vi "Glass Heater Accuracy.vi"() -> ()   [LabVIEW 2017]
uses:
  Shared Components/Gantry Class/Type Definitions/Virtual Modes.ctl
  Shared Components/Gantry Class/Type Definitions/Init_Modes.ctl
  Shared Components/Utils/Type Definitions/Object Types.ctl
  Shared Components/Config Manager Class/Type Definitions/Camera Enum.ctl
  Shared Components/Gantry Class/Gantry Class.lvclass
  Shared Components/Vec3d Class/Vec3d Class.lvclass
panel:
  in  "Results Folder":path=path "C:/Users/Admin/Gantry Purdue/pixel-gantry-control/Results"
  out "Iteration Number":i32
  in  "Virtual Mode":T1=enum."Virtual"
  in  "stop":bool
  out "Image":T2(plugin-control)
  out "error out":errorcluster
  in  "Config Folder":path=path "C:/Users/Admin/Gantry Purdue/pixel-gantry-control/Config"
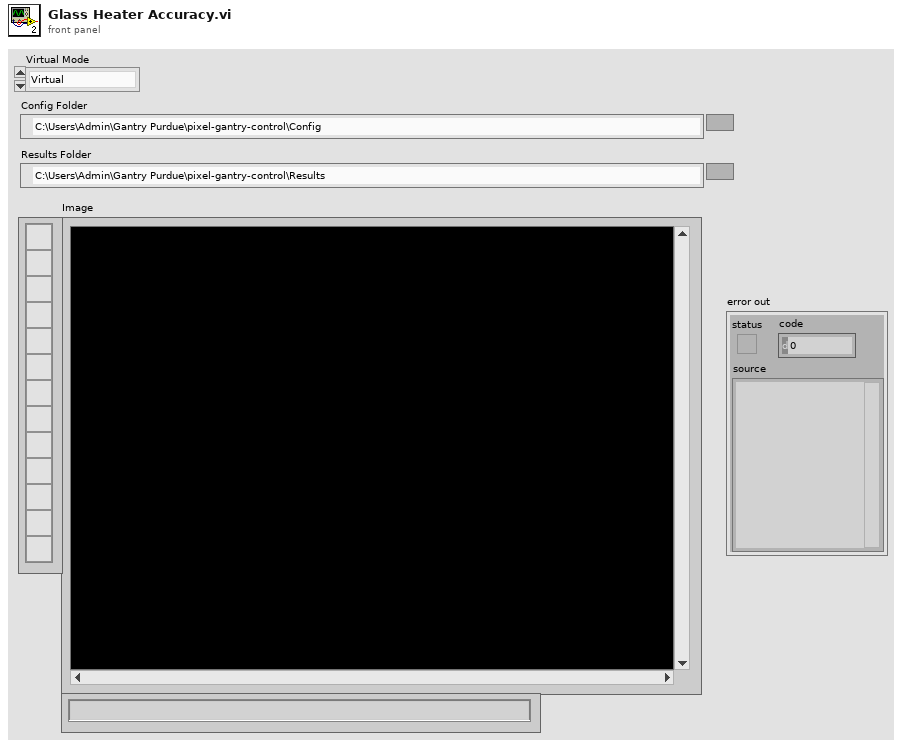
[diagram p1: front panel]
types:
  T1 = typedef "Virtual Modes.ctl" = enum16{"Nonvirtual", "Pseudovirtual", "Virtual"}
  T2 = typedef "IMAQ Image.ctl" = refnum<image>
  T3 = typedef "Init_Modes.ctl" = enum16{"Full", "Robot Only", "Dispenser Only", "Cameras Only", "Robot and Cameras", "Robot and Cameras and Dispenser", "Manifold Only"}
  T4 = typedef "Object Types.ctl" = enum16{"HDI", "Glass Piece", "Other"}
  T5 = typedef "Camera Enum.ctl" = enum16{"GANTRY HEAD", "NEEDLE CALIBRATION X", "NEEDLE CALIBRATION Y", "STAND CAMERA", "SIMRAN WEBCAM"}
  T6 = typedef "Physical Image.ctl" = cluster{"Image Position":refnum<class "Vec3d Class.lvclass">, "Image Reference":T2, "Field of View":cluster{"x(mm)":dbl, "y(mm)":dbl}}
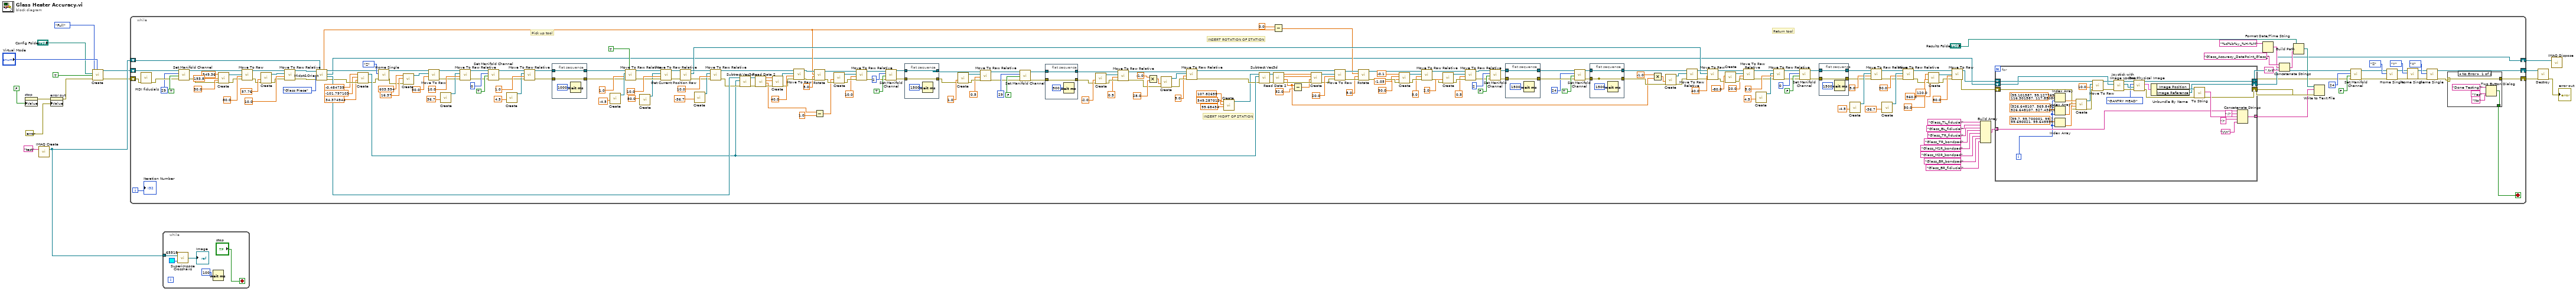
[diagram p0: block diagram]
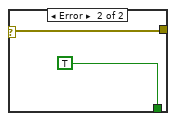
[diagram p2: hidden frame]
diagram:
  n1 = property on="stop" class="Bool (strict)"("Value"=FALSE) -> (error out=w14:errorcluster)  [unwired: 2 in, 1 out]
  n2 = call "IMAQ Create"("Image Name"="test") -> ("New Image"=w11:T2)  [unwired: 4 in, 1 out]
  n3 = property on="error out" class="Clust (strict)"(error in=w14, "Value"=errorcluster {"status"=FALSE, "code"=0, "source"=""} ("error in (no error)")) -> (error out=w9:errorcluster)  [unwired: 1 in, 1 out]
  n4 = call "Create.vi"("Virtual Mode"="Virtual Mode", "error in"=w9, "HOME?"=TRUE, "Config Folder"="Config Folder", "Init Mode"=Init_Modes."Full") -> ("error out"=w6:errorcluster, "Gantry out"=w5:refnum<class "Gantry Class.lvclass">)  [unwired: 5 in]
  n5 = while {
    shift-right: [w83] -> w3
    shift-left: w11 -> [w104]
    shift-right: [w106] -> w2
    shift-left: w5 -> [w140]
    shift-right: [w105] -> w1
    shift-left: w6 -> [w145]
    i -> [w142]
    stop <- w143 stop-if-true
    # "INSERT ROTATION OF STATION"
    # "INSERT MIDPT OF STATION"
    # "Pick up tool"
    # "Return tool"
    n6 = call "HDI fiducials"("error in (no error)"=w145) -> ("error out"=w138:errorcluster)  [unwired: 17 in, 1 out]
    n7 = call-dynamic "Set Manifold Channel.vi"("error in"=w138, "On/Off"=TRUE, "Manifold Channel"=29, "Gantry in"=w140) -> ("error out"=w137:errorcluster, "Gantry out"=w139:refnum<class "Gantry Class.lvclass">)  [unwired: 6 in]
    n8 = call "Create.vi"("error in"=w137, "Z"=30.0, "Y"=193.8, "X"=549.36) -> ("error out"=w225:errorcluster, "Vec3d Class out"=w258:refnum<class "Vec3d Class.lvclass">)  [unwired: 6 in]
    n9 = call-dynamic "Move To Raw.vi"("error in"=w225, "Speed"=80.0, "Destination"=w258, "Gantry in"=w139) -> ("error out"=w75:errorcluster, "Gantry out"=w80:refnum<class "Gantry Class.lvclass">)  [unwired: 6 in]
    n10 = call "Create.vi"("error in"=w75, "Z"=57.76) -> ("error out"=w74:errorcluster, "Vec3d Class out"=w81:refnum<class "Vec3d Class.lvclass">)  [unwired: 8 in]
    n11 = call-dynamic "Move To Raw Relative.vi"("error in"=w74, "Speed(mm/s)"=10.0, "Delta"=w81, "Gantry in"=w80) -> ("error out"=w78:errorcluster, "Gantry out"=w79:refnum<class "Gantry Class.lvclass">)  [unwired: 6 in]
    n12 = call-dynamic "Midpt&Orient.vi"("error in (no error)"=w78, "Enum"=Object_Types."Glass Piece", "Image In"=w104, "Gantry Class in"=w79) -> ("error out"=w158:errorcluster, "Midpoint"=w223:refnum<class "Vec3d Class.lvclass">, "Image Out"=w24:T2, "Gantry Class out"=w150:refnum<class "Gantry Class.lvclass">, "Orientation"=w147:dbl)  [unwired: 3 in]
    n13 = call "Create.vi"("error in"=w158, "Z"=34.374944 ("Y"), "Y"=-101.797103, "X"=-0.484739) -> ("error out"=w151:errorcluster, "Vec3d Class out"=w196:refnum<class "Vec3d Class.lvclass">)  [unwired: 6 in]
    n14 = call-dynamic "Home Single.vi"("error in"=w151, "Axis"=enum16{"X", "Y", "Z", "U"}."Z", "Gantry in"=w150) -> ("error out"=w148:errorcluster, "Gantry out"=w149:refnum<class "Gantry Class.lvclass">)  [unwired: 7 in]
    n15 = call "Create.vi"("error in"=w148, "Y"=16.37, "X"=603.594) -> ("Vec3d Class out"=w274:refnum<class "Vec3d Class.lvclass">)  [unwired: 7 in, 1 out]
    n16 = call-dynamic "Move To Raw.vi"("Speed"=50.0 ("Speed(mm/s)"), "Destination"=w274, "Gantry in"=w149) -> ("error out"=w170:errorcluster, "Gantry out"=w171:refnum<class "Gantry Class.lvclass">)  [unwired: 7 in]
    n17 = call "Create.vi"("Z"=36.7) -> ("Vec3d Class out"=w172:refnum<class "Vec3d Class.lvclass">)  [unwired: 9 in, 1 out]
    n18 = call-dynamic "Move To Raw Relative.vi"("error in"=w170, "Speed(mm/s)"=10.0, "Delta"=w172, "Gantry in"=w171) -> ("error out"=w64:errorcluster, "Gantry out"=w63:refnum<class "Gantry Class.lvclass">)  [unwired: 6 in]
    n19 = call-dynamic "Set Manifold Channel.vi"("error in"=w64, "On/Off"=TRUE, "Manifold Channel"=0, "Gantry in"=w63) -> ("error out"=w66:errorcluster, "Gantry out"=w68:refnum<class "Gantry Class.lvclass">)  [unwired: 6 in]
    n20 = call "Create.vi"("Z"=4.5) -> ("Vec3d Class out"=w69:refnum<class "Vec3d Class.lvclass">)  [unwired: 9 in, 1 out]
    n21 = call-dynamic "Move To Raw Relative.vi"("error in"=w66, "Speed(mm/s)"=1.0, "Delta"=w69, "Gantry in"=w68) -> ("error out"=w65:errorcluster, "Gantry out"=w67:refnum<class "Gantry Class.lvclass">)  [unwired: 6 in]
    n22 = flat-sequence {
      tunnel: w67 -> [w300]
      tunnel: [w300] -> w232
      tunnel: w65 -> [w298]
      tunnel: [w298] -> w231
      frame #0 {
        n23 = Wait (ms)(milliseconds to wait=u32 1000) -> ()  [unwired: 1 out]
      }
    }
    n24 = call "Create.vi"("Z"=-4.5) -> ("Vec3d Class out"=w269:refnum<class "Vec3d Class.lvclass">)  [unwired: 9 in, 1 out]
    n25 = call-dynamic "Move To Raw Relative.vi"("Wait?"=TRUE, "error in"=w231, "Speed(mm/s)"=1.0, "Delta"=w269, "Gantry in"=w232) -> ("error out"=w264:errorcluster, "Gantry out"=w265:refnum<class "Gantry Class.lvclass">)  [unwired: 5 in]
    n26 = call "Create.vi"("Y"=80.0 ("Z")) -> ("Vec3d Class out"=w263:refnum<class "Vec3d Class.lvclass">)  [unwired: 9 in, 1 out]
    n27 = call-dynamic "Move To Raw Relative.vi"("error in"=w264, "Speed(mm/s)"=10.0, "Delta"=w263, "Gantry in"=w265) -> ("error out"=w251:errorcluster, "Gantry out"=w253:refnum<class "Gantry Class.lvclass">)  [unwired: 6 in]
    n28 = call-dynamic "Get Current Position Raw.vi"("error in"=w251, "Gantry in"=w253) -> ("error out"=w250:errorcluster, "Vec3d Class out"=w187:refnum<class "Vec3d Class.lvclass">, "Gantry out"=w252:refnum<class "Gantry Class.lvclass">)  [unwired: 7 in]
    n29 = call "Create.vi"("Z"=-36.7) -> ("Vec3d Class out"=w259:refnum<class "Vec3d Class.lvclass">)  [unwired: 9 in, 1 out]
    n30 = call-dynamic "Move To Raw Relative.vi"("error in"=w250, "Speed(mm/s)"=10.0, "Delta"=w259, "Gantry in"=w252) -> ("error out"=w217:errorcluster, "Gantry out"=w215:refnum<class "Gantry Class.lvclass">)  [unwired: 6 in]
    n31 = call "Subtract Vec3d.vi"("error in (no error)"=w217, "Vec3d in 2"=w196, "Vec3d in 1"=w223) -> ("error out"=w219:errorcluster, "Vec3d Class out"=w176:refnum<class "Vec3d Class.lvclass">)  [unwired: 7 in]
    n32 = call-dynamic "Read Data 2.vi"("error in"=w219, "Vec3d in"=w176) -> ("error out"=w218:errorcluster, "Z"=w51:dbl, "Y"=w221:dbl, "X"=w222:dbl)  [unwired: 6 in]
    n33 = call "Create.vi"("error in"=w218, "Y"=w221, "X"=w222) -> ("error out"=w216:errorcluster, "Vec3d Class out"=w175:refnum<class "Vec3d Class.lvclass">)  [unwired: 7 in]
    n34 = call-dynamic "Move To Raw.vi"("error in"=w216, "Speed"=40.0, "Destination"=w175, "Gantry in"=w215) -> ("error out"=w186:errorcluster, "Gantry out"=w185:refnum<class "Gantry Class.lvclass">)  [unwired: 6 in]
    n35 = call-dynamic "Rotate.vi"("error in"=w186, "speed(deg/s)"=5.0, "distance(deg)"=w147, "Gantry in"=w185) -> ("error out"=w183:errorcluster, "Gantry out"=w184:refnum<class "Gantry Class.lvclass">)  [unwired: 6 in]
    n36 = Subtract(x=w51, y=1.0) -> (x-y=w50:dbl)
    n37 = call "Create.vi"("error in"=w183, "Z"=w50) -> ("error out"=w214:errorcluster, "Vec3d Class out"=w220:refnum<class "Vec3d Class.lvclass">)  [unwired: 8 in]
    n38 = call-dynamic "Move To Raw Relative.vi"("error in"=w214, "Speed(mm/s)"=10.0, "Delta"=w220, "Gantry in"=w184) -> ("error out"=w58:errorcluster, "Gantry out"=w57:refnum<class "Gantry Class.lvclass">)  [unwired: 6 in]
    n39 = call-dynamic "Set Manifold Channel.vi"("error in"=w58, "On/Off"=TRUE, "Manifold Channel"=2, "Gantry in"=w57) -> ("error out"=w60:errorcluster, "Gantry out"=w61:refnum<class "Gantry Class.lvclass">)  [unwired: 6 in]
    n40 = flat-sequence {
      tunnel: w61 -> [w278]
      tunnel: [w278] -> w53
      tunnel: w60 -> [w276]
      tunnel: [w276] -> w46
      frame #0 {
        n41 = Wait (ms)(milliseconds to wait=u32 1500) -> ()  [unwired: 1 out]
      }
    }
    n42 = call "Create.vi"("error in"=w46, "Z"=1.0 ("y")) -> ("error out"=w55:errorcluster, "Vec3d Class out"=w56:refnum<class "Vec3d Class.lvclass">)  [unwired: 8 in]
    n43 = call-dynamic "Move To Raw Relative.vi"("error in"=w55, "Speed(mm/s)"=0.5, "Delta"=w56, "Gantry in"=w53) -> ("error out"=w47:errorcluster, "Gantry out"=w48:refnum<class "Gantry Class.lvclass">)  [unwired: 6 in]
    n44 = call-dynamic "Set Manifold Channel.vi"("error in"=w47, "On/Off"=FALSE, "Manifold Channel"=29, "Gantry in"=w48) -> ("error out"=w133:errorcluster, "Gantry out"=w132:refnum<class "Gantry Class.lvclass">)  [unwired: 6 in]
    n45 = flat-sequence {
      tunnel: w132 -> [w284]
      tunnel: [w284] -> w41
      tunnel: w133 -> [w282]
      tunnel: [w282] -> w40
      frame #0 {
        n46 = Wait (ms)(milliseconds to wait=u32 500) -> ()  [unwired: 1 out]
      }
    }
    n47 = call "Create.vi"("error in"=w40, "Z"=-2.0 ("y")) -> ("error out"=w44:errorcluster, "Vec3d Class out"=w45:refnum<class "Vec3d Class.lvclass">)  [unwired: 8 in]
    n48 = call-dynamic "Move To Raw Relative.vi"("error in"=w44, "Speed(mm/s)"=0.5, "Delta"=w45, "Gantry in"=w41) -> ("error out"=w38:errorcluster, "Gantry out"=w39:refnum<class "Gantry Class.lvclass">)  [unwired: 6 in]
    n49 = Multiply(x=-1.0, y=28.0) -> (x*y=w256:dbl)
    n50 = call "Create.vi"("error in"=w38, "Z"=w256) -> ("error out"=w254:errorcluster, "Vec3d Class out"=w255:refnum<class "Vec3d Class.lvclass">)  [unwired: 8 in]
    n51 = call-dynamic "Move To Raw Relative.vi"("error in"=w254, "Speed(mm/s)"=5.0, "Delta"=w255, "Gantry in"=w39) -> ("error out"=w192:errorcluster, "Gantry out"=w193:refnum<class "Gantry Class.lvclass">)  [unwired: 6 in]
    n52 = call "Create.vi"("Z"=99.68434, "Y"=549.287012, "X"=107.82655) -> ("Vec3d Class out"=w103:refnum<class "Vec3d Class.lvclass">)  [unwired: 7 in, 1 out]
    n53 = call "Subtract Vec3d.vi"("error in (no error)"=w192, "Vec3d in 2"=w196, "Vec3d in 1"=w103) -> ("error out"=w203:errorcluster, "Vec3d Class out"=w206:refnum<class "Vec3d Class.lvclass">)  [unwired: 7 in]
    n54 = Subtract(x=0.0, y=w147) -> (x-y=w146:dbl)
    n55 = call-dynamic "Read Data 2.vi"("error in"=w203, "Vec3d in"=w206) -> ("error out"=w202:errorcluster, "Z"=w94:dbl, "Y"=w207:dbl, "X"=w208:dbl)  [unwired: 6 in]
    n56 = Subtract(x=w94, y=32.0) -> (x-y=w93:dbl)
    n57 = call "Create.vi"("error in"=w202, "Z"=w93, "Y"=w207, "X"=w208) -> ("error out"=w201:errorcluster, "Vec3d Class out"=w205:refnum<class "Vec3d Class.lvclass">)  [unwired: 6 in]
    n58 = call-dynamic "Move To Raw.vi"("error in"=w201, "Speed"=20.0, "Destination"=w205, "Gantry in"=w193) -> ("error out"=w180:errorcluster, "Gantry out"=w181:refnum<class "Gantry Class.lvclass">)  [unwired: 6 in]
    n59 = call-dynamic "Rotate.vi"("error in"=w180, "speed(deg/s)"=5.0, "distance(deg)"=w146, "Gantry in"=w181) -> ("error out"=w179:errorcluster, "Gantry out"=w178:refnum<class "Gantry Class.lvclass">)  [unwired: 6 in]
    n60 = call "Create.vi"("error in"=w179, "Z"=30.0, "Y"=-1.05, "X"=-0.1) -> ("error out"=w200:errorcluster, "Vec3d Class out"=w204:refnum<class "Vec3d Class.lvclass">)  [unwired: 6 in]
    n61 = call-dynamic "Move To Raw Relative.vi"("error in"=w200, "Speed(mm/s)"=5.0, "Delta"=w204, "Gantry in"=w178) -> ("error out"=w32:errorcluster, "Gantry out"=w33:refnum<class "Gantry Class.lvclass">)  [unwired: 6 in]
    n62 = call "Create.vi"("error in"=w32, "Z"=2.0) -> ("error out"=w36:errorcluster, "Vec3d Class out"=w37:refnum<class "Vec3d Class.lvclass">)  [unwired: 8 in]
    n63 = call-dynamic "Move To Raw Relative.vi"("error in"=w36, "Speed(mm/s)"=0.5, "Delta"=w37, "Gantry in"=w33) -> ("error out"=w31:errorcluster, "Gantry out"=w30:refnum<class "Gantry Class.lvclass">)  [unwired: 6 in]
    n64 = call-dynamic "Set Manifold Channel.vi"("error in"=w31, "On/Off"=FALSE, "Manifold Channel"=2, "Gantry in"=w30) -> ("error out"=w195:errorcluster, "Gantry out"=w194:refnum<class "Gantry Class.lvclass">)  [unwired: 6 in]
    n65 = flat-sequence {
      tunnel: w194 -> [w294]
      tunnel: [w294] -> w128
      tunnel: w195 -> [w292]
      tunnel: [w292] -> w125
      frame #0 {
        n66 = Wait (ms)(milliseconds to wait=u32 1500) -> ()  [unwired: 1 out]
      }
    }
    n67 = call-dynamic "Set Manifold Channel.vi"("error in"=w125, "On/Off"=TRUE, "Manifold Channel"=24, "Gantry in"=w128) -> ("error out"=w130:errorcluster, "Gantry out"=w129:refnum<class "Gantry Class.lvclass">)  [unwired: 6 in]
    n68 = flat-sequence {
      tunnel: w129 -> [w281]
      tunnel: [w281] -> w127
      tunnel: w130 -> [w279]
      tunnel: [w279] -> _
      tunnel: [w279] -> w126
      frame #0 {
        n69 = Wait (ms)(milliseconds to wait=u32 1500) -> ()  [unwired: 1 out]
      }
    }
    n70 = Multiply(x=-1.0, y=w94) -> (x*y=w210:dbl)
    n71 = call "Create.vi"("error in"=w126, "Z"=w210) -> ("error out"=w191:errorcluster, "Vec3d Class out"=w188:refnum<class "Vec3d Class.lvclass">)  [unwired: 8 in]
    n72 = call-dynamic "Move To Raw Relative.vi"("error in"=w191, "Delta"=w188, "Gantry in"=w127) -> ("error out"=w189:errorcluster, "Gantry out"=w190:refnum<class "Gantry Class.lvclass">)  [unwired: 7 in]
    n73 = call-dynamic "Move To Raw.vi"("error in"=w189, "Speed"=40.0, "Destination"=w187, "Gantry in"=w190) -> ("error out"=w161:errorcluster, "Gantry out"=w169:refnum<class "Gantry Class.lvclass">)  [unwired: 6 in]
    n74 = call "Create.vi"("error in"=w161, "Y"=-80.0) -> ("error out"=w248:errorcluster, "Vec3d Class out"=w233:refnum<class "Vec3d Class.lvclass">)  [unwired: 8 in]
    n75 = call-dynamic "Move To Raw Relative.vi"("error in"=w248, "Speed(mm/s)"=20.0, "Delta"=w233, "Gantry in"=w169) -> ("error out"=w234:errorcluster, "Gantry out"=w235:refnum<class "Gantry Class.lvclass">)  [unwired: 6 in]
    n76 = call "Create.vi"("Z"=4.5) -> ("Vec3d Class out"=w241:refnum<class "Vec3d Class.lvclass">)  [unwired: 9 in, 1 out]
    n77 = call-dynamic "Move To Raw Relative.vi"("error in"=w234, "Speed(mm/s)"=5.0, "Delta"=w241, "Gantry in"=w235) -> ("error out"=w239:errorcluster, "Gantry out"=w240:refnum<class "Gantry Class.lvclass">)  [unwired: 6 in]
    n78 = call-dynamic "Set Manifold Channel.vi"("error in"=w239, "On/Off"=FALSE, "Manifold Channel"=0, "Gantry in"=w240) -> ("error out"=w228:errorcluster, "Gantry out"=w230:refnum<class "Gantry Class.lvclass">)  [unwired: 6 in]
    n79 = flat-sequence {
      tunnel: w230 -> [w297]
      tunnel: [w297] -> w229
      tunnel: w228 -> [w295]
      tunnel: [w295] -> w227
      frame #0 {
        n80 = Wait (ms)(milliseconds to wait=u32 1500) -> ()  [unwired: 1 out]
      }
    }
    n81 = call "Create.vi"("Z"=-4.5) -> ("Vec3d Class out"=w237:refnum<class "Vec3d Class.lvclass">)  [unwired: 9 in, 1 out]
    n82 = call-dynamic "Move To Raw Relative.vi"("error in"=w227, "Speed(mm/s)"=5.0, "Delta"=w237, "Gantry in"=w229) -> ("error out"=w116:errorcluster, "Gantry out"=w117:refnum<class "Gantry Class.lvclass">)  [unwired: 6 in]
    n83 = call "Create.vi"("Z"=-36.7) -> ("Vec3d Class out"=w119:refnum<class "Vec3d Class.lvclass">)  [unwired: 9 in, 1 out]
    n84 = call-dynamic "Move To Raw Relative.vi"("error in"=w116, "Speed(mm/s)"=50.0, "Delta"=w119, "Gantry in"=w117) -> ("error out"=w107:errorcluster, "Gantry out"=w108:refnum<class "Gantry Class.lvclass">)  [unwired: 6 in]
    n85 = call "Create.vi"("error in"=w107, "Z"=30.0, "Y"=560.0, "X"=120.0) -> ("error out"=w111:errorcluster, "Vec3d Class out"=w113:refnum<class "Vec3d Class.lvclass">)  [unwired: 6 in]
    n86 = call-dynamic "Move To Raw.vi"("error in"=w111, "Speed"=80.0, "Destination"=w113, "Gantry in"=w108) -> ("error out"=w25:errorcluster, "Gantry out"=w26:refnum<class "Gantry Class.lvclass">)  [unwired: 6 in]
    n87 = Build Array("Glass_TL_fiducial" ("string"), "Glass_BL_fidiucial" ("string"), "Glass_TR_fiducial" ("string"), "Glass_TR_bondpad" ("string"), "Glass_M1R_bondpad" ("string"), "Glass_M2R_bondpad" ("string"), "Glass_BR_bondpad" ("string"), "Glass_BR_fidiucial" ("string")) -> (w27:string[])
    n88 = for {
      tunnel: [w324] -> w23 mode=indexing
      shift-right: [w325] -> w85
      shift-left: w25 -> [w301]
      shift-right: [w323] -> w84
      shift-left: w26 -> [w318]
      shift-right: [w319] -> w83
      shift-left: w24 -> [w307]
      tunnel: w27 -> [w303] mode=indexing
      i -> [w302]
      n89 = Index Array(array=dbl[] [99.101587, 99.127769, 116.301587, 117.850807, 117.863228, 117.862293, 117.873652, 116.327769], index=w302) -> (element=w315:dbl)
      n90 = Index Array(array=dbl[] [526.648107, 569.84924, 526.648107, 527.43622, 547.203352, 549.29103, 569.056008, 569.84924], index=w302) -> (element=w314:dbl)
      n91 = Index Array(array=dbl[] [99.7, 99.700001, 99.7, 99.690021, 99.649999, 99.684328, 99.645157, 99.700001], index=w302) -> (element=w305:dbl)
      n92 = call "Create.vi"("error in"=w301, "Z"=w305, "Y"=w314, "X"=w315) -> ("error out"=w312:errorcluster, "Vec3d Class out"=w313:refnum<class "Vec3d Class.lvclass">)  [unwired: 6 in]
      n93 = call-dynamic "Move To Raw.vi"("error in"=w312, "Speed"=10.0, "Destination"=w313, "Gantry in"=w318) -> ("error out"=w317:errorcluster, "Gantry out"=w316:refnum<class "Gantry Class.lvclass">)  [unwired: 6 in]
      n94 = call-dynamic "Joystick with Image Update.vi"("error in (no error)"=w317, "Image In"=w307, "Gantry Class in"=w316) -> ("error out"=w331:errorcluster, "Image Out"=w322:T2, "Gantry Class out"=w330:refnum<class "Gantry Class.lvclass">)  [unwired: 6 in]
      n95 = call-dynamic "Get Physical Image.vi"("error in"=w331, "Image In"=w322, "Camera Name"=Camera_Enum."GANTRY HEAD", "Gantry in"=w330) -> ("error out"=w304:errorcluster, "Physical Image"=w329:T6, "Gantry out"=w323:refnum<class "Gantry Class.lvclass">)  [unwired: 5 in]
      n96 = Unbundle By Name(w329) -> ("Image Position"=w328:refnum<class "Vec3d Class.lvclass">, "Image Reference"=w319:T2)
      n97 = call "To String.vi"("error in"=w304, "Vec3d in"=w328) -> ("error out"=w325:errorcluster, "Vec3d String"=w326:string)  [unwired: 7 in, 1 out]
      n98 = Concatenate Strings(w303, ":(" ("string"), w326, ")" ("string"), "\r\n" ("string")) -> (w324:string)
    }
    n99 = Format Date/Time String(time format string (%c)="%d%b%y_%H-%M") -> (date/time string=w86:string)  [unwired: 2 in]
    n100 = Concatenate Strings("Glass_Accuracy_DataPoint_Glass_" ("name or relative path"), w86, ".txt" ("string")) -> (w88:string)
    n101 = Build Path(base path="Results Folder", name or relative path=w88) -> (appended path=w91:path)
    n102 = Write to Text File(file (use dialog)=w91, text=w23, error in=w85) -> (error out=w82:errorcluster)  [unwired: 1 in, 2 out]
    n103 = call-dynamic "Set Manifold Channel.vi"("error in"=w82, "On/Off"=FALSE, "Manifold Channel"=24, "Gantry in"=w84) -> ("error out"=w121:errorcluster, "Gantry out"=w120:refnum<class "Gantry Class.lvclass">)  [unwired: 6 in]
    n104 = call-dynamic "Home Single.vi"("error in"=w121, "Axis"=enum16{"X", "Y", "Z", "U"}."Z", "Gantry in"=w120) -> ("error out"=w164:errorcluster, "Gantry out"=w165:refnum<class "Gantry Class.lvclass">)  [unwired: 7 in]
    n105 = call-dynamic "Home Single.vi"("error in"=w164, "Axis"=enum16{"X", "Y", "Z", "U"}."Y", "Gantry in"=w165) -> ("error out"=w162:errorcluster, "Gantry out"=w163:refnum<class "Gantry Class.lvclass">)  [unwired: 7 in]
    n106 = call-dynamic "Home Single.vi"("error in"=w162, "Axis"=enum16{"X", "Y", "Z", "U"}."X", "Gantry in"=w163) -> ("error out"=w144:errorcluster, "Gantry out"=w106:refnum<class "Gantry Class.lvclass">)  [unwired: 7 in]
    n107 = case shown="No Error" w144 {
      selector: w144 -> [w285 w291]
      tunnel: [w285 w291] -> w105
      tunnel: [w286 TRUE ("Done Testing?")] -> w143
      frame No Error {
        n108 = Two Button Dialog(message="Done Testing?", 1:"No" ("F button name (\"Cancel\")"), 2:"Yes" ("T button name (\"OK\")")) -> (T button?=w286:bool)
      }
      frame Error {
      }
    }
    "Iteration Number" <- w142
  }
  n109 = while {
    tunnel: w11 -> [w334]
    stop <- "stop" stop-if-true
    n110 = call "Superimpose Crosshairs.vi"("Grid Line Color"=u32 65518, "Refnum in"=w334) -> ("Refnum out"=→"Image":T2)
    n111 = Wait (ms)(milliseconds to wait=u32 100) -> ()  [unwired: 1 out]
  }
  n112 = call "Destroy.vi"("error in"=w1, "Gantry Class in"=w2) -> ("error out"=→"error out":errorcluster)  [unwired: 9 in]
  n113 = call "IMAQ Dispose"("Image"=w3) -> ()  [unwired: 5 in, 1 out]
